vi "Gripper.vi"(4 "Side":T1, 8 "error in":errorcluster, 10 "Open?":bool caption="Open", 11 "Target Position":sgl) -> (0 "error out":errorcluster, 3 "On Target":bool)   [LabVIEW 2013]
uses:
  ROS/Code/SubVIs/BaxterSide.ctl
panel:
  in  "Threshold":sgl=10.0
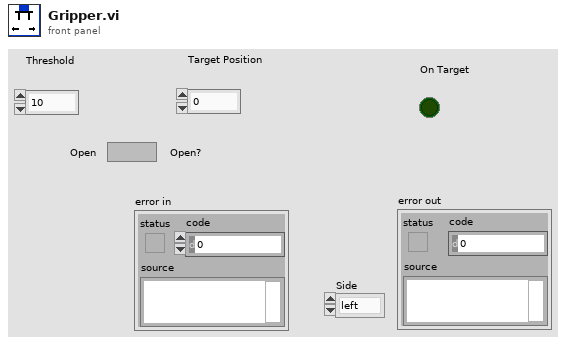
[diagram p1: front panel]
types:
  T1 = typedef "BaxterSide.ctl" = enum16{"left", "right"}
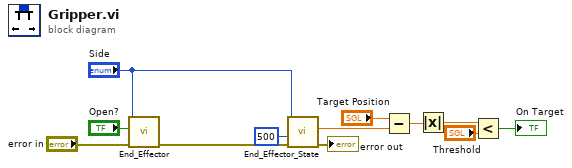
[diagram p0: block diagram]
diagram:
  n1 = call "End_Effector.vi"("error in"="error in", "Close"="Open?", "Side"="Side") -> ("error out"=w10:errorcluster)  [unwired: 5 in]
  n2 = call "End_Effector_State.vi"("error in"=w10, "Delay"=u32 500, "Side"="Side") -> ("error out"=→"error out":errorcluster, "position"=w7:sgl)  [unwired: 2 in, 2 out]
  n3 = Subtract(x="Target Position", y=w7) -> (x-y=w4:sgl)
  n4 = Absolute Value(x=w4) -> (abs(x)=w3:sgl)
  n5 = Less?(x=w3, y="Threshold") -> (x < y?=→"On Target":bool)
